vi "7.3.1.vi"() -> ()   [LabVIEW 2018]
panel:
  in  "c":string
  in  "b":string
  in  "a":bool
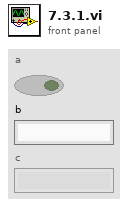
[diagram p1: front panel]
types:
  T1 = enum8{"Enabled", "Disabled", "Disabled and Grayed Out"}
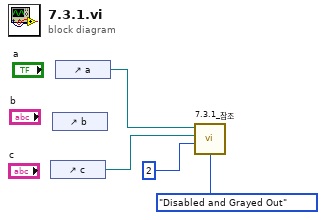
[diagram p0: block diagram]
diagram:
  n1 = control-ref of="c"() -> (w1:refnum<vi>)
  n2 = control-ref of="b"() -> ()  [unwired: 1 out]
  n3 = control-ref of="a"() -> (w4:refnum<vi>)
  n4 = call "7.3.1_참조.vi"("비활성화"=T1."Disabled and Grayed Out", "디스플레이 스타일"=u32 2, "Str 참조 번호"=w1, "Bool 참조 번호"=w4) -> ()
